vi "Write timeouts.vi"(8 "error in (no error)":errorcluster, 10 "MB timeouts":T1={"reconn_timeout"=3000, "N attempt max"=3, "t_reset_TTL"=120000, "period"=100} {"t_reset_TTL" min=10 max=240000 step=1; "period" min=10 max=100000 step=1; "N attempt max" min=1 max=5 step=1; "reconn_timeout" min=10 max=240000 step=1}, 11 "MB_TCP in":refnum<class "Modbus Master CR.lvclass">) -> (0 "error out":errorcluster, 3 "MB_TCP out":refnum<class "Modbus Master CR.lvclass">)   [LabVIEW 2021, in "Modbus Master CR.lvclass"]
uses:
  Modbus Master CR.lvclass
  ctl/MB timeouts.ctl
  Modbus Master CR.lvclass/Modbus Master CR.ctl
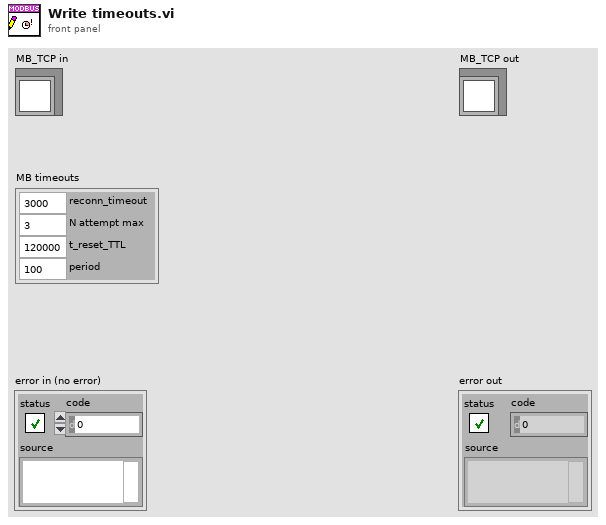
[diagram p1: front panel]
types:
  T1 = typedef "Modbus Master CR.lvclass/MB timeouts.ctl" = cluster{"reconn_timeout":i32, "N attempt max":i32, "t_reset_TTL":i32, "period":i32}
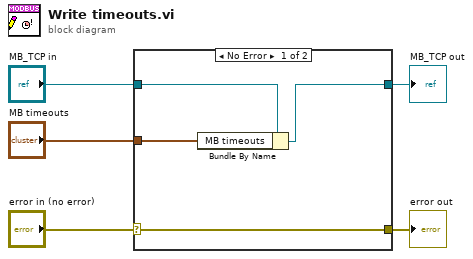
[diagram p0: block diagram]
diagram:
  n1 = case shown="No Error" "error in (no error)" {
    selector: "error in (no error)" -> [w6 w10]
    tunnel: [w6 w10] -> w4
    tunnel: [w8 w11] -> w2
    tunnel: "MB_TCP in" -> [w7 w11]
    tunnel: "MB timeouts" -> [w9 _]
    frame No Error {
      n2 = Bundle By Name(cluster=w7, "MB timeouts"=w9) -> (w8:refnum<class "Modbus Master CR.lvclass">)
    }
    frame Error {
    }
  }
  "error out" <- w4
  "MB_TCP out" <- w2
